vi "Initialise.vi"(8 "error in (no error)":errorcluster, 9 "Include Container Name with Tag":bool, 10 "SV Container":refnum<k21>, 11 "SharedVariable_Bus in":refnum<class "SharedVariable_Bus.lvclass">) -> (0 "error out":errorcluster, 3 "SharedVariable_Bus out":refnum<class "SharedVariable_Bus.lvclass">)   [LabVIEW 2021, in "SharedVariable_Bus.lvclass"]
uses:
  SharedVariable_Bus.lvclass
  C:/Program Files (x86)/National Instruments/LabVIEW 2021/vi.lib/TSA/Omni-Bus/Omni-Bus/Bus Access/Bus_Access.lvclass
  SharedVariable_Bus.lvclass/SharedVariable_Bus.ctl
  <vilib>/TSA/Omni-Bus/Omni-Bus/Bus Access/Bus_Access.lvclass/Bus_Access.ctl
  Properties/Write SV Containers.vi
  <vilib>/TSA/Omni-Bus/Omni-Bus/Bus Access/Properties/Write Tag Root.vi
  Properties/Write Add Container Name to Tag.vi
panel:
  in  "Tag Root":string
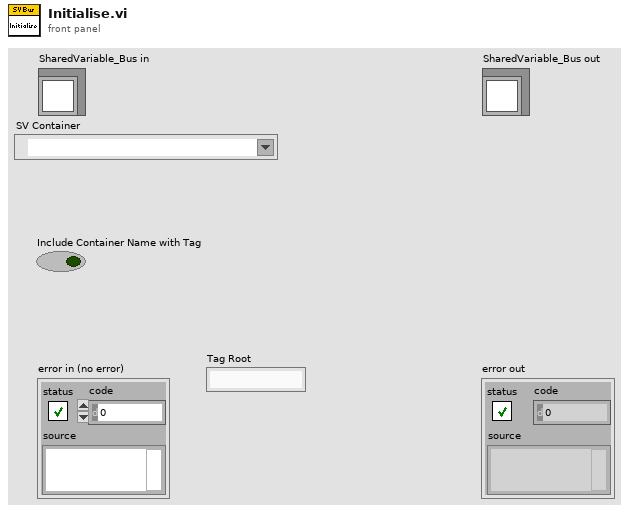
[diagram p1: front panel]
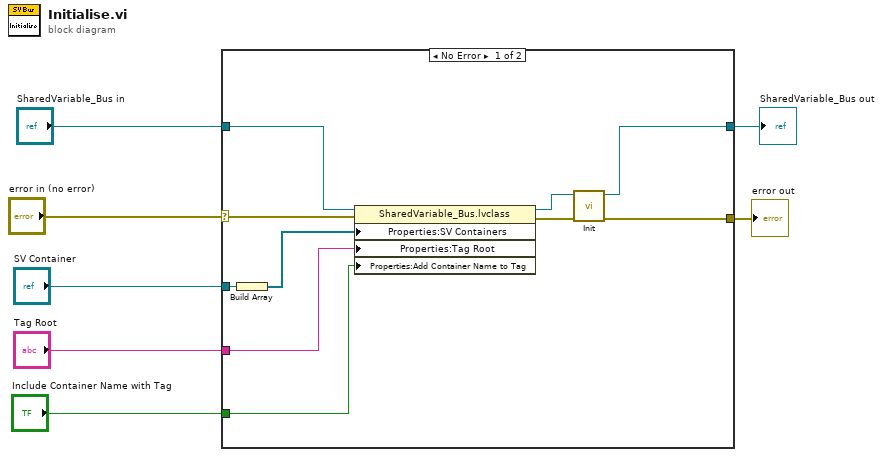
[diagram p0: block diagram]
diagram:
  n1 = case shown="No Error" "error in (no error)" {
    selector: "error in (no error)" -> [w17 w19]
    tunnel: [w14 w19] -> w6
    tunnel: [w12 w18] -> w4
    tunnel: "SharedVariable_Bus in" -> [w16 w18]
    tunnel: "SV Container" -> [w11 _]
    tunnel: "Tag Root" -> [w10 _]
    tunnel: "Include Container Name with Tag" -> [w8 _]
    frame No Error {
      n2 = Build Array(w11) -> (w9:refnum<k21>[])
      n3 = property class="SharedVariable_Bus.lvclass"(reference=w16, error in=w17, "Properties:SV Containers"=w9, "Properties:Tag Root"=w10, "Properties:Add Container Name to Tag"=w8) -> (reference out=w13:refnum<class "SharedVariable_Bus.lvclass">, error out=w15:errorcluster)
      n4 = call-dynamic "Init.vi"("error in (no error)"=w15, "Data in"=w13) -> ("error out"=w14:errorcluster, "Data out"=w12:refnum<class "SharedVariable_Bus.lvclass">)  [unwired: 8 in]
    }
    frame Error {
    }
  }
  "error out" <- w6
  "SharedVariable_Bus out" <- w4
